vi "Get Config File.vi"() -> (0 "error out":errorcluster, 3 "File Path Control":path)   [LabVIEW 2019, in "Topas.lvlib"]
uses:
  Topas.lvlib
  <vilib>/Utility/config.llb/Read Key (String).vi
  <vilib>/Utility/config.llb/NI_LVConfig.lvlib
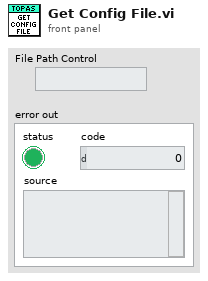
[diagram p1: front panel]
types:
  T1 = typedef "NI_LVConfig.lvlib/Config Data RefNum.ctl" = refnum<k1>
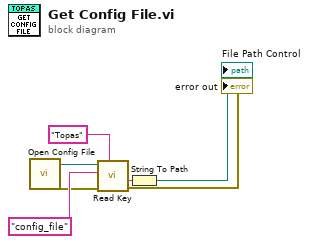
[diagram p0: block diagram]
diagram:
  n1 = call "Open Config File.vi"() -> ("error out"=w2:errorcluster, "Refnum out"=w1:T1)  [unwired: 10 in]
  n2 = call-poly <vilib>:"Read Key.vi"("section"="Topas", "error in (no error)"=w2, "key"="config_file", "refnum"=w1) -> ("error out"=→"error out":errorcluster, "value"=w3:string)  [unwired: 4 in, 2 out]
  n3 = String To Path(string=w3) -> (path=→"File Path Control":path)
